vi "T 1 (SubVI).vi"(10 "arg":dbl format="%#_13g") -> (2 "matrix":dbl[][](array[numeric]))   [LabVIEW 2017]
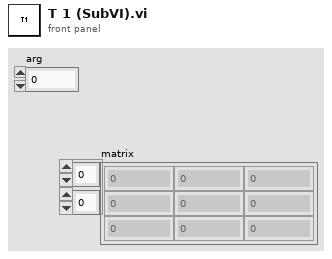
[diagram p1: front panel]
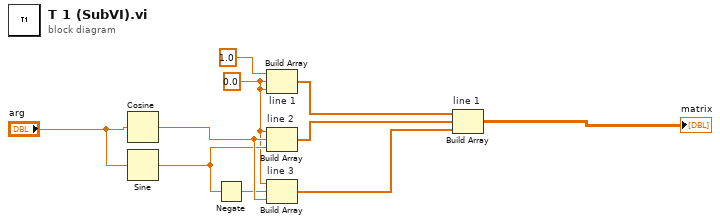
[diagram p0: block diagram]
diagram:
  w7 = 0.0 ("element")
  n1 = Cosine(x="arg") -> (cos(x)=w10:dbl)
  n2 = Sine(x="arg") -> (sin(x)=w9:dbl)
  n3 = Negate(x=w9) -> (-x=w8:dbl)
  n4 = Build Array "line 1"(1.0 ("element"), w7, w7) -> (w2:dbl[])
  n5 = Build Array "line 2"(w7, w10, w9) -> (w3:dbl[])
  n6 = Build Array "line 3"(w7, w8, w10) -> (w4:dbl[])
  n7 = Build Array "line 1"(w2, w3, w4) -> (→"matrix":dbl[][])
